vi "SEND_INICIARG.vi"(8 "error in (no error)":errorcluster, 10 "GUARDAR?":bool, 11 "GUARDADOTEXTOPLANO in":refnum<class "GUARDADOTEXTOPLANO.lvclass">) -> (0 "error out":errorcluster, 3 "GUARDADOTEXTOPLANO out":refnum<class "GUARDADOTEXTOPLANO.lvclass">)   [LabVIEW 2019, in "GUARDADOTEXTOPLANO.lvlib" / "GUARDADOTEXTOPLANO.lvclass"]
uses:
  GUARDADOTEXTOPLANO.lvclass
  GUARDADOTEXTOPLANO.lvclass/GUARDADOTEXTOPLANO.ctl
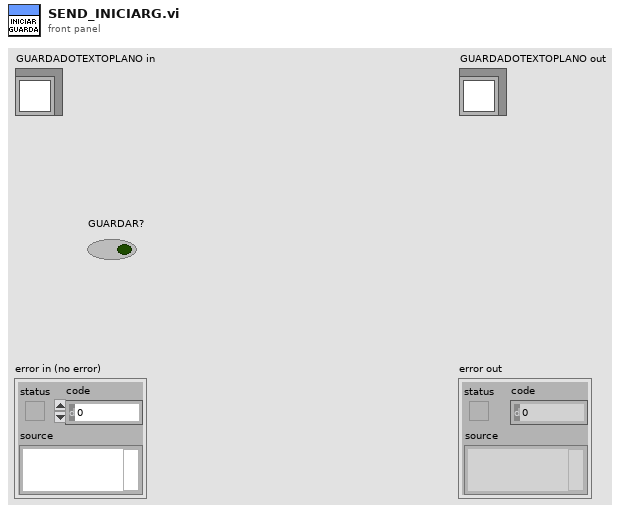
[diagram p1: front panel]
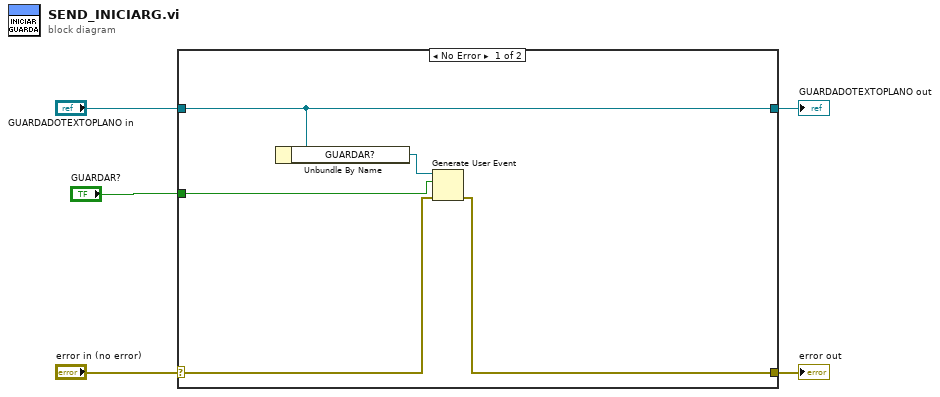
[diagram p0: block diagram]
diagram:
  n1 = case shown="No Error" "error in (no error)" {
    selector: "error in (no error)" -> [w7 w12]
    tunnel: [w6 w12] -> w4
    tunnel: [w10 w11] -> w2
    tunnel: "GUARDADOTEXTOPLANO in" -> [w10 w11]
    tunnel: "GUARDAR?" -> [w8 _]
    frame No Error {
      n2 = Unbundle By Name(w10) -> ("GUARDAR?"=w9:refnum<user-event>)
      n3 = Generate User Event(user event=w9, event data cluster=w8, error in=w7) -> (error out=w6:errorcluster)  [unwired: 1 in, 1 out]
    }
    frame Error {
    }
  }
  "error out" <- w4
  "GUARDADOTEXTOPLANO out" <- w2
